vi "Read Rule parser.vi"(9 "Selection":string, 11 "UIManager in":refnum<class "UIManager.lvclass">) -> (1 "Parameters":string, 2 "IRuleFileParser.lvclass":refnum<class "IRuleFileParser.lvclass">, 3 "UIManager out":refnum<class "UIManager.lvclass">, 4 "found?":bool)   [LabVIEW 2020, in "DependencyInspector.lvlib" / "UIManager.lvclass"]
uses:
  UIManager.lvclass
  ExtensionInterfaces/IRuleFileParser/IRuleFileParser.lvclass
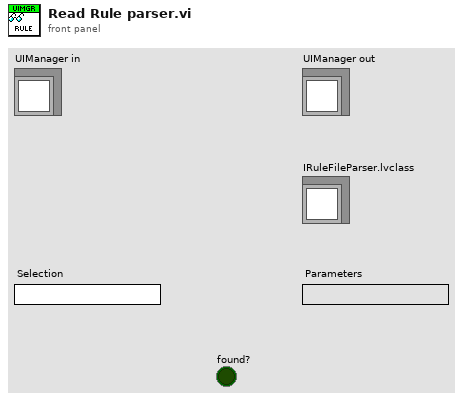
[diagram p1: front panel]
types:
  T1 = map{string, refnum<class "IRuleFileParser.lvclass">}
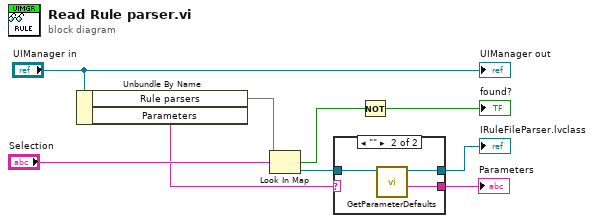
[diagram p0: block diagram]
diagram:
  n1 = Unbundle By Name("UIManager in") -> ("Rule parsers"=w7:T1, "Parameters"=w4:string)
  n2 = Look In Map(map=w7, key="Selection") -> (key not found?=w6:bool, value=w2:refnum<class "IRuleFileParser.lvclass">)  [unwired: 1 in]
  n3 = case shown="\"\"" w4 {
    selector: w4 -> [w11 _]
    tunnel: [w11 w13] -> w3
    tunnel: w2 -> [w10 w14]
    tunnel: [w10 w12] -> w1
    frame Default {
    }
    frame "" {
      n4 = call-dynamic "GetParameterDefaults.vi"("IRuleFileParser in"=w14) -> ("Parameter defaults"=w13:string, "IRuleFileParser out"=w12:refnum<class "IRuleFileParser.lvclass">)  [unwired: 8 in, 1 out]
    }
  }
  "IRuleFileParser.lvclass" <- w1
  "Parameters" <- w3
  n5 = Not(x=w6) -> (.not. x?=→"found?":bool)
  "UIManager out" <- "UIManager in"
